vi "Write TDMS.vi"(8 "error in (no error)":errorcluster, 9 "Gyros Data":T1, 10 "Accelerometer Data":T2, 11 "Sparkfun Atomic IMU in":refnum<class "Sparkfun Atomic IMU.lvclass">) -> (0 "error out":errorcluster, 3 "Sparkfun Atomic IMU out":refnum<class "Sparkfun Atomic IMU.lvclass">)   [LabVIEW 2019, in "Sparkfun Atomic IMU.lvclass"]
doc: "Writes data to the tdms file. Call Open TDMS VI before running this VI."
uses:
  Sparkfun Atomic IMU.lvclass
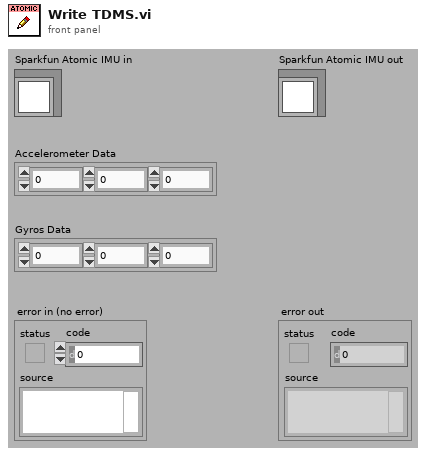
[diagram p1: front panel]
types:
  T1 = cluster{"Pitch (deg/s)":dbl, "Roll (deg/s)":dbl, "Yaw (deg/s)":dbl}
  T2 = cluster{"Accel_X (g)":dbl, "Accel_Y (g)":dbl, "Accel_Z (g)":dbl}
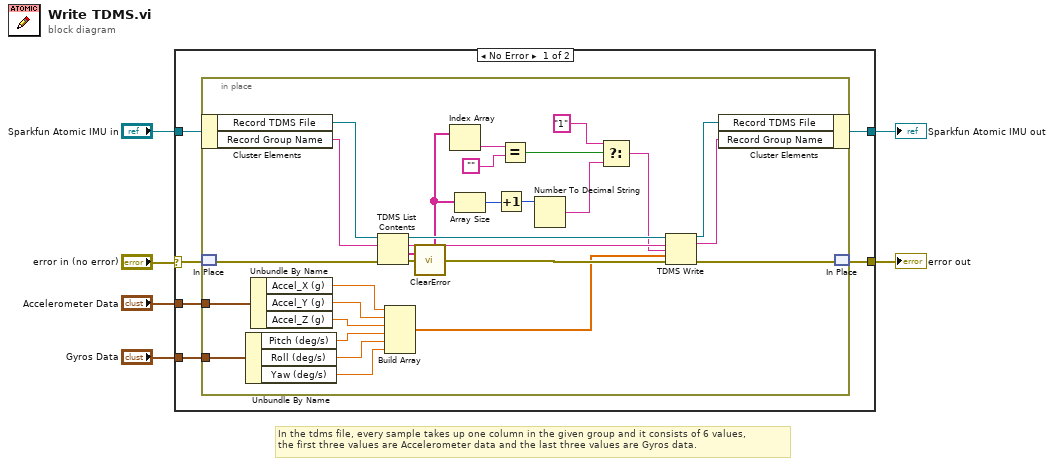
[diagram p0: block diagram]
diagram:
  # "In the tdms file, every sample takes up one column in the given group and it consists of 6 values, \nthe first three values are Accelerometer data and the last three values are Gyros data."
  n1 = case shown="No Error" "error in (no error)" {
    selector: "error in (no error)" -> [w11 w42]
    tunnel: "Sparkfun Atomic IMU in" -> [w12 w41]
    tunnel: [w10 w42] -> w4
    tunnel: [w9 w41] -> w3
    tunnel: "Accelerometer Data" -> [w8 _]
    tunnel: "Gyros Data" -> [w7 _]
    frame No Error {
      n2 = in-place {
        in-place-border: w8 -> [w23]
        in-place-border: w7 -> [w22]
        n3 = in-place-cluster #1(w12) -> ("Record TDMS File"=w40:refnum<k34>, "Record Group Name"=w32:string)
        n4 = in-place-match #2(w11) -> (w33:errorcluster)
        n5 = Unbundle By Name(w22) -> ("Pitch (deg/s)"=w18:dbl, "Roll (deg/s)"=w17:dbl, "Yaw (deg/s)"=w16:dbl)
        n6 = Unbundle By Name(w23) -> ("Accel_X (g)"=w21:dbl, "Accel_Y (g)"=w20:dbl, "Accel_Z (g)"=w19:dbl)
        n7 = TDMS List Contents(4:w33, 6:w32, 7:w40) -> (0:w13:errorcluster, 1:w27:string[], 2:w30:string, 3:w31:refnum<k34>)
        n8 = Build Array(w21, w20, w19, w18, w17, w16) -> (w15:dbl[])
        n9 = call <vilib>:"ClearError.vi"("error in (no error)"=w13) -> ("error out"=w28:errorcluster)
        n10 = Index Array(array=w27) -> (element=w39:string)  [unwired: 1 in]
        n11 = Array Size(array=w27) -> (size(s)=w35:i32)
        n12 = Increment(x=w35) -> (x+1=w34:i32)
        n13 = Equal?(x=w39, y="") -> (x = y?=w37:bool)
        n14 = Number To Decimal String(number=w34) -> (decimal integer string=w29:string)  [unwired: 1 in]
        n15 = Select(t="1", s=w37, f=w29) -> (s? t:f=w14:string)
        n16 = TDMS Write(0:w31, 5:w30, 7:w14, 9:w15, 11:w28) -> (4:w26:refnum<k34>, 6:w25:string, 15:w24:errorcluster)  [unwired: 1 in, 1 out]
        n17 = in-place-cluster #1("Record TDMS File"=w26, "Record Group Name"=w25) -> (w9:refnum<class "Sparkfun Atomic IMU.lvclass">)
        n18 = in-place-match #2(w24) -> (w10:errorcluster)
      }
    }
    frame Error {
    }
  }
  "Sparkfun Atomic IMU out" <- w3
  "error out" <- w4
